vi "GetTickCount.vi"(5 "error in (no error)":errorcluster={"status"=FALSE, "code"=1073676294, "source"="VISA Read in CONEC-CC.lvclass:WriteReadSerialPort.vi->CONEC-CC.lvclass:Get Motion Time.vi->Stage Control 01.vi"}) -> (16 "ms":u32, 19 "error IO":errorcluster={"status"=FALSE, "code"=1073676294, "source"="VISA Read in CONEC-CC.lvclass:WriteReadSerialPort.vi->CONEC-CC.lvclass:Get Motion Time.vi->Stage Control 01.vi"})   [LabVIEW 2018]
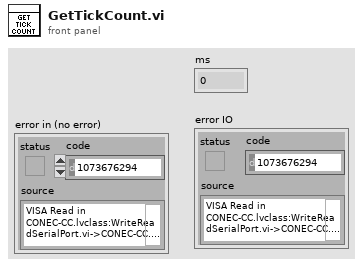
[diagram p1: front panel]
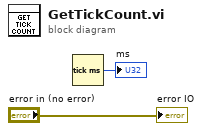
[diagram p0: block diagram]
diagram:
  n1 = Tick Count (ms)() -> (millisecond timer value=→"ms":u32)
  "error IO" <- "error in (no error)"
